vi "1-Parallel Resistors.vi"() -> ()   [LabVIEW 2014]
panel:
  out "Equivalent Resistance":dbl format="%#_3g"
  in  "Resistance 2":dbl
  in  "Resistance 1":dbl
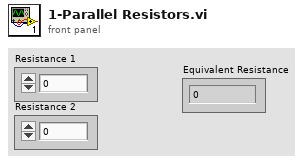
[diagram p1: front panel]
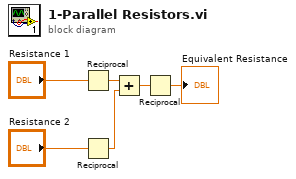
[diagram p0: block diagram]
diagram:
  n1 = Reciprocal(x="Resistance 1") -> (1/x=w3:dbl)
  n2 = Reciprocal(x="Resistance 2") -> (1/x=w4:dbl)
  n3 = Add(x=w3, y=w4) -> (x+y=w2:dbl)
  n4 = Reciprocal(x=w2) -> (1/x=→"Equivalent Resistance":dbl)
